vi "SaveDataFile.vi"(1 "Temperature":dbl, 2 "Run uninterrupted?":bool, 3 "Humidity":dbl, 7 "Sensor Index/\nSegment No.":u32, 11 "Error In":errorcluster, 12 "Array Titles":string, 13 "Strip Segment":string) -> (4 "Filename OUT":string, 8 "Pathname OUT":string, 10 "Path + Filename OUT":string, 15 "Error Out":errorcluster)   [LabVIEW 2018]
uses:
  globals/QC_RunInformation.vi
panel:
  out "File header":string
  out "File name":string
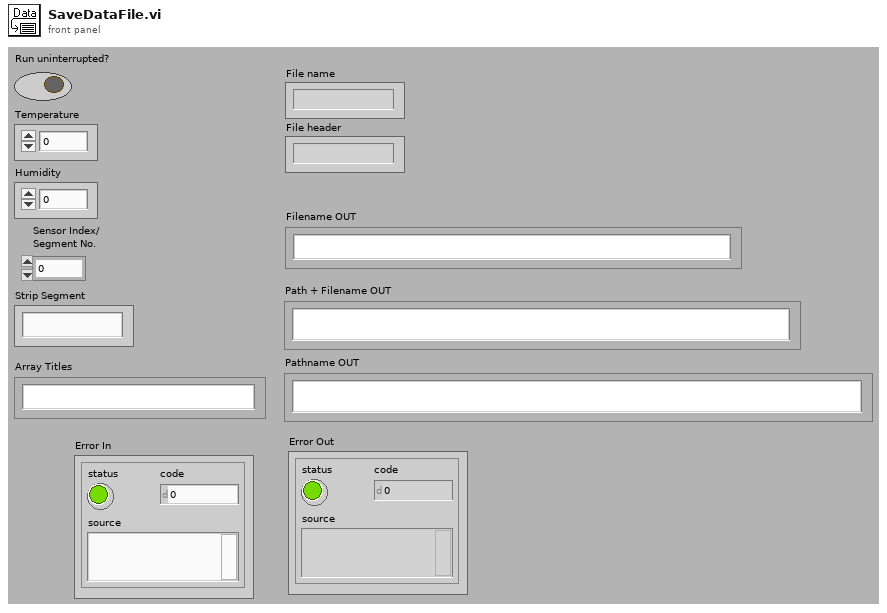
[diagram p1: front panel]
types:
  T1 = enum16{"open", "open or create", "create or replace", "create"}
  T2 = cluster{"Sensor Serial No.:":string, "Wafer:":string, "Batch:":string, "Manufacturer:":string, "Device Category:":string, "Database Serial No.:":string, "Date Initiated:":string, "Time Initiated:":string, "Test":string, "Probeplan used:":string, "End of Run Status":dbl, "End of Run comment:":string, "User:":string, "Vbias SMU":string, "LCR":string, "Test SMU":string, "Test DMM":string, "Comments":string, "Measurement results":cluster{"IV":string, "CV":string, "Cis":string, "Ris":string, "Stability":string, "PTP":string, "Striptest":string}}
  T3 = cluster{"Institute":string, "Manufacturers":string[], "Devices":string[], "Serialnumbers Lookup DB":string, "Data directory":string, "Backup & screenshot directory":string, "List of known users":string[], "Measurement switch not used":bool, "Measurement Switch":string, "DUT Switch":string, "Rseries IV [MOhm]":string, "Rshunt IV [MOhm]":string, "Rseries CV [MOhm]":string, "DC blocking Cap [µF]":string, "Rseries LCR [MOhm]":string, "Rseries stability [MOhm]":string, "Rshunt stability [MOhm]":string, "Rseries striptest bias [MOhm]":string, "Rseries strip pinhole [MOhm]":string}
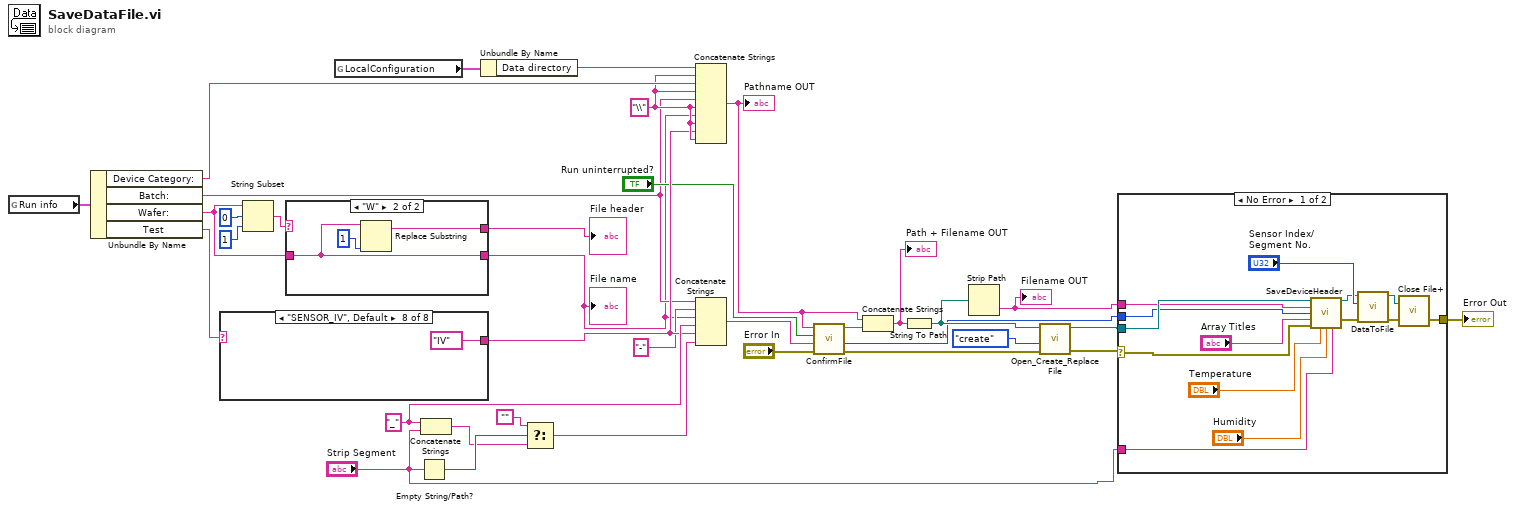
[diagram p0: block diagram]
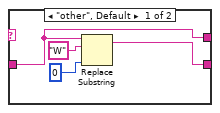
[diagram p2: hidden frame]
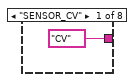
[diagram p3: hidden frame]
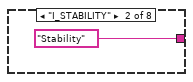
[diagram p4: hidden frame]
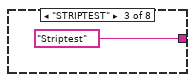
[diagram p5: hidden frame]
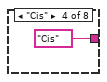
[diagram p6: hidden frame]
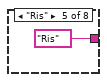
[diagram p7: hidden frame]
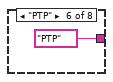
[diagram p8: hidden frame]
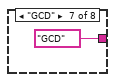
[diagram p9: hidden frame]
diagram:
  w19 = "_"
  w28 = "\\"
  n1 = global read "QC_RunInformation.vi" "Run info"() -> (w33:T2)
  n2 = Unbundle By Name(w33) -> ("Device Category:"=w31:string, "Batch:"=w13:string, "Wafer:"=w6:string, "Test"=w16:string)
  n3 = case shown="\"SENSOR_IV\", Default" w16 {
    tunnel: ["CV" ("Test") "Stability" ("Test") "Striptest" ("Test") "Cis" ("Test") "Ris" ("Test") "PTP" ("Test") "GCD" ("Test") "IV" ("Test")] -> w15
    frame "SENSOR_CV" {
    }
    frame "I_STABILITY" {
    }
    frame "STRIPTEST" {
    }
    frame "Cis" {
    }
    frame "Ris" {
    }
    frame "PTP" {
    }
    frame "GCD" {
    }
    frame "SENSOR_IV", Default {
    }
  }
  n4 = String Subset(string=w6, offset (0)=0, length (rest)=1 ("length (rest)")) -> (substring=w9:string)
  n5 = case shown="\"W\"" w9 {
    tunnel: [w45 w49] -> w7
    tunnel: w6 -> [w44 w49]
    tunnel: [w44 w50] -> w8
    frame "other", Default {
      n6 = Replace Substring(2:0 ("length (len. of substring)"), 4:"W" ("substring (\"\")"), 5:w44) -> (1:w45:string)  [unwired: 1 in, 1 out]
    }
    frame "W" {
      n7 = Replace Substring(2:1 ("length (len. of substring)"), 5:w49) -> (1:w50:string)  [unwired: 2 in, 1 out]
    }
  }
  "File name" <- w7
  "File header" <- w8
  n8 = global read "QC_RunInformation.vi" "LocalConfiguration"() -> (w34:T3)
  n9 = Empty String/Path?(string/path="Strip Segment") -> (empty?=w21:bool)
  n10 = Concatenate Strings(w19, "Strip Segment") -> (w17:string)
  n11 = Unbundle By Name(w34) -> ("Data directory"=w32:string)
  n12 = Select(t="", s=w21, f=w17) -> (s? t:f=w18:string)
  n13 = Concatenate Strings(w32, w28, w31, w28, w13, w28, w7, w28, w15, w28) -> (w24:string)
  "Pathname OUT" <- w24
  n14 = Concatenate Strings(w13, "-" ("string"), w7, w19, w15, w18) -> (w27:string)
  n15 = call "ConfirmFile.vi"("Error In"="Error In", "Filename IN"=w27, "Run uninterrupted?"="Run uninterrupted?", "Pathname IN"=w24) -> ("Error Out"=w25:errorcluster, "Run Number"=w2:i32, "Filename:"=w23:string)  [unwired: 1 in]
  n16 = Concatenate Strings(w24, w23) -> (w22:string)
  "Path + Filename OUT" <- w22
  n17 = String To Path(string=w22) -> (path=w29:path)
  n18 = Strip Path(path=w29) -> (name=w1:string)  [unwired: 1 out]
  "Filename OUT" <- w1
  n19 = call <vilib>:"Open_Create_Replace File.vi"("error in (no error)"=w25, "function (open:0)"=T1."create", "file path"=w29) -> ("error out"=w4:errorcluster, "refnum"=w3:refnum<file>)  [unwired: 5 in, 2 out]
  n20 = case shown="No Error" w4 {
    selector: w4 -> [w64 w65]
    tunnel: w3 -> [w63 _]
    tunnel: w1 -> [w62 _]
    tunnel: [w60 w65] -> w35
    tunnel: w2 -> [w57 _]
    tunnel: "Strip Segment" -> [w56 _]
    frame No Error {
      n21 = call "SaveDeviceHeader.vi"("File Refnum in"=w63, "Filename"=w62, "Run Number"=w57, "Array Titles"="Array Titles", "error in (no error)"=w64, "Temperature"="Temperature", "Humidity"="Humidity", "Strip Segment"=w56) -> ("File Refnum out"=w54:refnum<file>, "error out"=w53:errorcluster)  [unwired: 5 in, 1 out]
      n22 = call "DataToFile.vi"("error in (no error)"=w53, "Sensor Index/\nSegment No."="Sensor Index/\nSegment No.", "File Refnum in"=w54) -> ("error out"=w52:errorcluster, "File Refnum out"=w51:refnum<file>)  [unwired: 7 in]
      n23 = call <vilib>:"Close File+.vi"("error in (no error)"=w52, "refnum"=w51) -> ("error out"=w60:errorcluster)  [unwired: 3 in, 2 out]
    }
    frame Error {
    }
  }
  "Error Out" <- w35
